vi "Test MQTT-3.1.2-18.vi"(8 "error in (no error)":errorcluster) -> (0 "error out":errorcluster)   [LabVIEW 2013]
uses:
  source/Control Packets/CONNECT/ConnectFlags -- cluster.ctl
  <vilib>/addons/_JKI Toolkits/Caraya/classes/Assert/Assert Error.vi
  source/Control Packets/CONNECT/CONNECT.lvclass
  <vilib>/addons/_JKI Toolkits/Caraya/classes/Test/Test.lvclass
  <vilib>/addons/_JKI Toolkits/Caraya/classes/Assert/Assert.lvclass
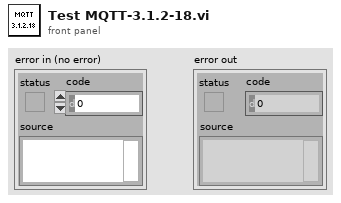
[diagram p1: front panel]
types:
  T1 = cluster{"Will Topic":string, "Will Message":string, "Username":string, "Password":string}
  T2 = typedef "CONNECT.lvclass/ConnectFlags -- cluster.ctl" = cluster{"Reserved":bool, "Clean Session":bool, "Will Flag":bool, "Will QoS 1":bool, "Will QoS 2":bool, "Will Retain":bool, "Password Flag":bool, "User Name Flag":bool}
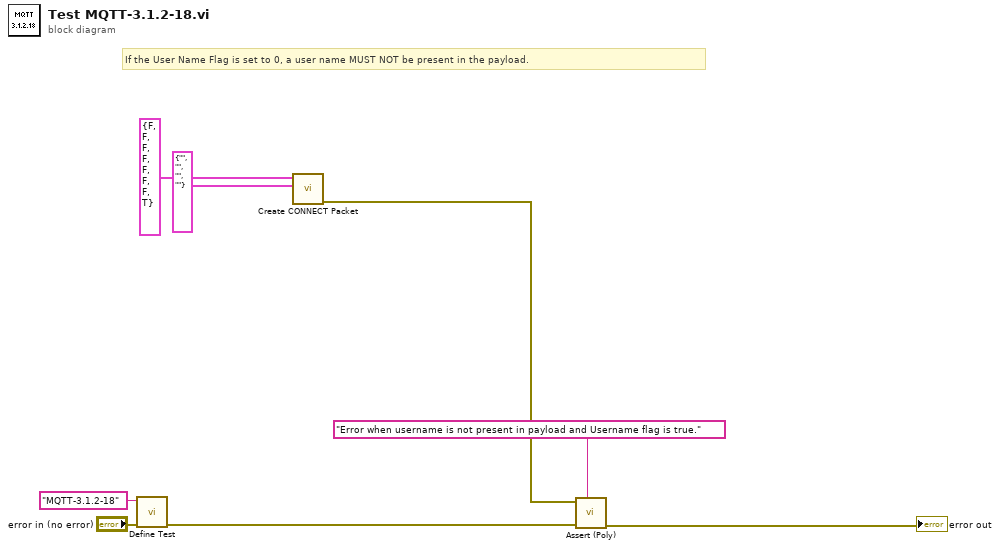
[diagram p0: block diagram]
diagram:
  # "If the User Name Flag is set to 0, a user name MUST NOT be present in the payload."
  n1 = call <vilib>:"Define Test.vi"("error in (no error)"="error in (no error)", "Label (VI Title)"="MQTT-3.1.2-18") -> ("error out"=w1:errorcluster)  [unwired: 9 in]
  n2 = call "Create CONNECT Packet.vi"("Payload"=T1 {"Will Topic"="", "Will Message"="", "Username"="", "Password"=""}, "Connect Flags"=T2 {"Reserved"=FALSE, "Clean Session"=FALSE, "Will Flag"=FALSE, "Will QoS 1"=FALSE, "Will QoS 2"=FALSE, "Will Retain"=FALSE, "Password Flag"=FALSE, "User Name Flag"=TRUE}) -> ("error out"=w4:errorcluster)  [unwired: 8 in, 1 out]
  n3 = call-poly <vilib>:"Assert (Poly).vi"("Label"="Error when username is not present in payload and Username flag is true.", "error in (no error)"=w1, "Error?"=w4) -> ("error out"=→"error out":errorcluster)  [unwired: 8 in]
